vi "HEWH Start Index Check.vi"(6 "Energy (BTU) Index":i32, 9 "Test Start Index":i32, 10 "Full Data w/o Information Header in":dbl[][](array[numeric]) format="%#_6f", 11 "Time Column Index":i32) -> (1 "Energy (BTU) Index out":i32, 2 "Test Start Index  (Full Index) out":i32)   [LabVIEW 2023]
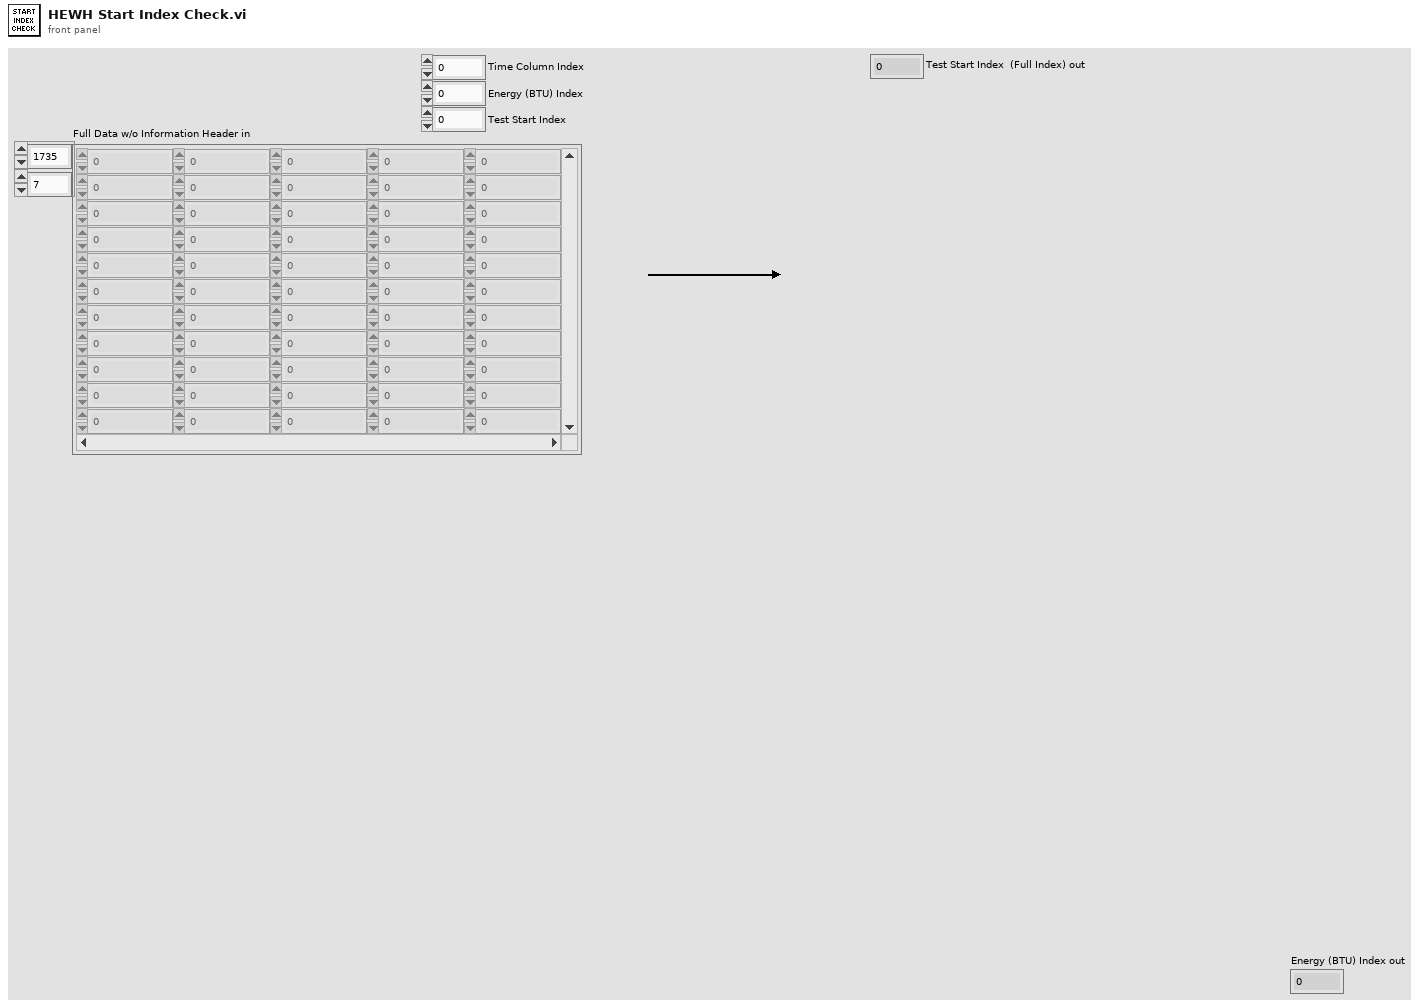
[diagram p1: front panel]
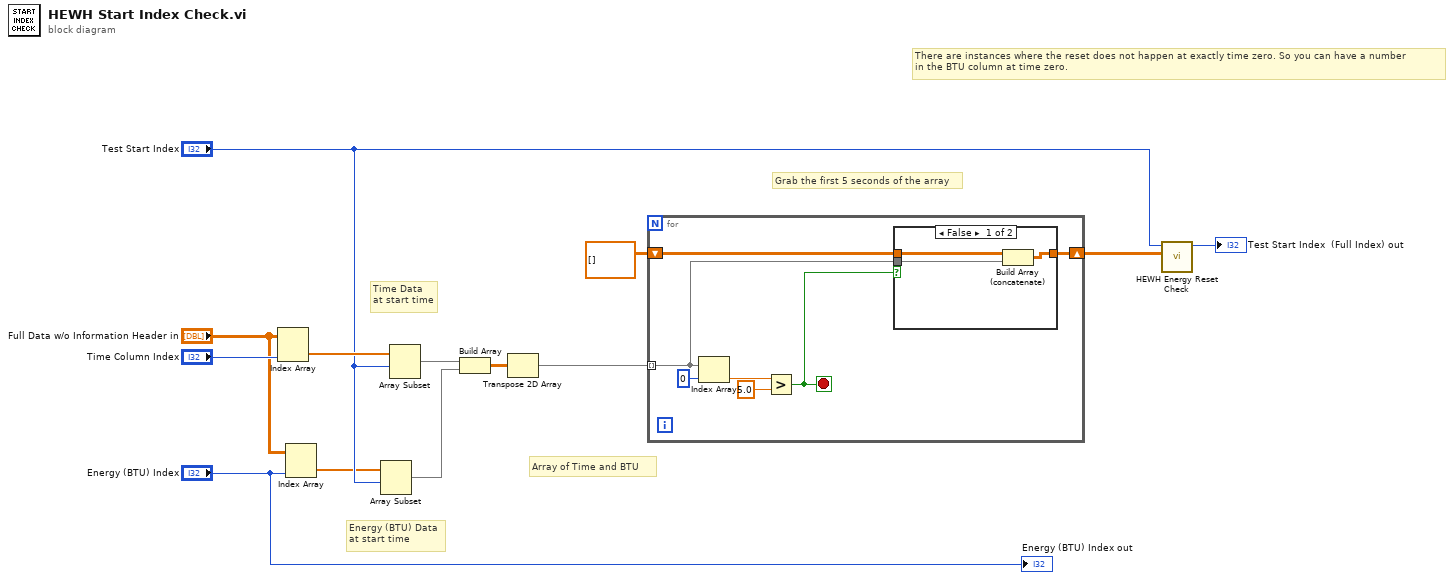
[diagram p0: block diagram]
diagram:
  # "There are instances where the reset does not happen at exactly time zero. So you can have a number \nin the BTU column at time zero."
  # "Array of Time and BTU"
  # "Grab the first 5 seconds of the array"
  # "Energy (BTU) Data\nat start time"
  # "Time Data\nat start time"
  n1 = Index Array(array="Full Data w/o Information Header in", index (col)="Time Column Index") -> (element=w10:dbl[])  [unwired: 1 in]
  n2 = Index Array(array="Full Data w/o Information Header in", index (col)="Energy (BTU) Index") -> (element=w6:dbl[])  [unwired: 1 in]
  n3 = Array Subset(array=w6, index="Test Start Index") -> (w12:dbl[])  [unwired: 1 in]
  n4 = Array Subset(array=w10, index="Test Start Index") -> (w11:dbl[])  [unwired: 1 in]
  n5 = Build Array(w11, w12) -> (w13:dbl[][])
  n6 = Transpose 2D Array(2D array=w13) -> (transposed array=w3:dbl[][])
  n7 = for {
    tunnel: w3 -> [w15] mode=indexing
    shift-right: [w19] -> w2
    shift-left: dbl[][] [] -> [w20]
    stop <- w14 stop-if-true
    n8 = Index Array(array=w15, index=0) -> (element=w17:dbl)
    n9 = Greater?(x=w17, y=5.0) -> (0:w14:bool)
    n10 = case shown="False" w14 {
      tunnel: w20 -> [w23 w24]
      tunnel: [w22 w24] -> w19
      tunnel: w15 -> [w21 _]
      frame False {
        n11 = Build Array (concatenate)(w23, w21) -> (w22:dbl[][])
      }
      frame True {
      }
    }
  }
  n12 = call "HEWH Energy Reset Check.vi"("Input Data"=w2, "Test Start Index"="Test Start Index") -> ("Test Start Index  (Full Index) out"=→"Test Start Index  (Full Index) out":i32)  [unwired: 8 in, 1 out]
  "Energy (BTU) Index out" <- "Energy (BTU) Index"
